vi "Query Device ID.vi"(0 "DMM in":refnum<class "DMM.lvclass">, 11 "error in (no error)":errorcluster) -> (4 "DMM out":refnum<class "DMM.lvclass">, 6 "Model":string, 8 "Serial Number":string, 10 "Firmware":string, 15 "error out":errorcluster)   [LabVIEW 2018, in "DMM.lvlib" / "DMM.lvclass"]
uses:
  DMM.lvclass
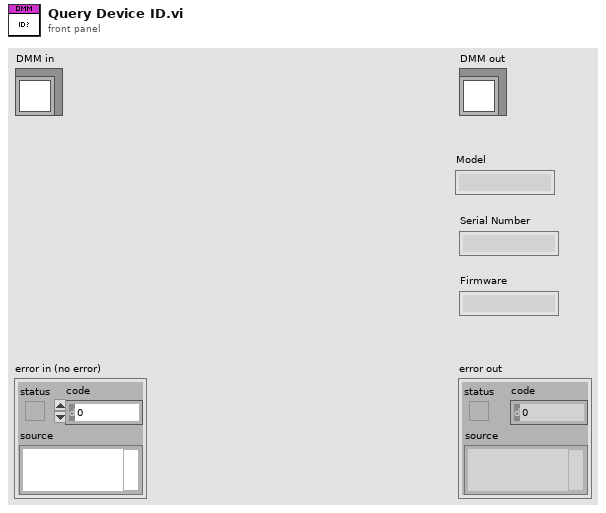
[diagram p1: front panel]
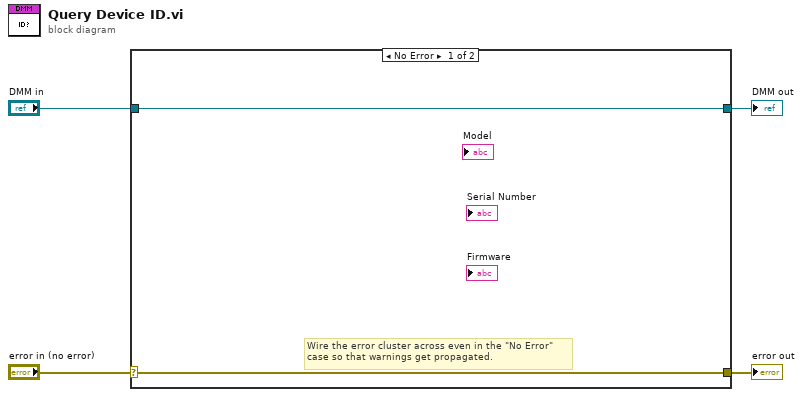
[diagram p0: block diagram]
diagram:
  n1 = case shown="No Error" "error in (no error)" {
    selector: "error in (no error)" -> [w5 w8]
    tunnel: [w5 w8] -> w3
    tunnel: [w6 w7] -> w1
    tunnel: "DMM in" -> [w6 w7]
    frame No Error {
      # "Wire the error cluster across even in the \"No Error\"\ncase so that warnings get propagated."
    }
    frame Error {
    }
  }
  "error out" <- w3
  "DMM out" <- w1
